vi "Read Keys.vi"(7 "Section":string, 8 "error in (no error)":errorcluster, 10 "Key Names ([]=All Keys)":string[](array[string]), 11 "Config Refnum in":T1) -> (0 "error out":errorcluster, 1 "Values":string[](array[string]), 2 "Key Names":string[](array[string]), 3 "Config Refnum out":T1, 4 "Found":bool[](array[boolean]))   [LabVIEW 2018, in "Core.lvlib" / "Config.lvlib"]
uses:
  Config.lvlib
  <vilib>/Utility/config.llb/NI_LVConfig.lvlib
  <vilib>/Utility/config.llb/Read Key (String).vi
  <vilib>/Utility/config.llb/Config Data RefNum.ctl
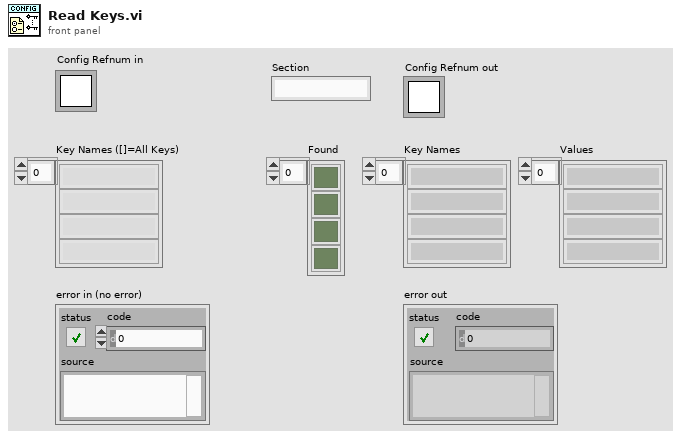
[diagram p1: front panel]
types:
  T1 = typedef "NI_LVConfig.lvlib/Config Data RefNum.ctl" = refnum<k1>
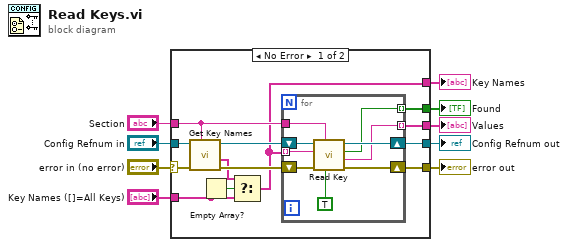
[diagram p0: block diagram]
diagram:
  n1 = case shown="No Error" "error in (no error)" {
    selector: "error in (no error)" -> [w12 w33]
    tunnel: "Section" -> [w20 _]
    tunnel: [w11 w33] -> w7
    tunnel: [w19 _] -> w6
    tunnel: [w18 _] -> w5
    tunnel: "Key Names ([]=All Keys)" -> [w16 _]
    tunnel: [w14 _] -> w3
    tunnel: "Config Refnum in" -> [w13 w32]
    tunnel: [w10 w32] -> w1
    frame No Error {
      n2 = call <vilib>:"Get Key Names.vi"("section"=w20, "error in (no error)"=w12, "refnum"=w13) -> ("error out"=w22:errorcluster, "key names"=w15:string[], "refnum out"=w21:T1)  [unwired: 5 in, 1 out]
      n3 = Empty Array?(array=w16) -> (empty?=w17:bool)
      n4 = Select(t=w15, s=w17, f=w16) -> (s? t:f=w14:string[])
      n5 = for {
        shift-right: [w28] -> w11
        shift-left: w22 -> [w31]
        shift-right: [w29] -> w10
        shift-left: w21 -> [w30]
        tunnel: w14 -> [w26] mode=indexing
        tunnel: w20 -> [w25]
        tunnel: [w24] -> w19 mode=indexing
        tunnel: [w23] -> w18 mode=indexing
        n6 = call-poly <vilib>:"Read Key.vi"("read raw string? (F)"=TRUE, "section"=w25, "error in (no error)"=w31, "key"=w26, "refnum"=w30) -> ("error out"=w28:errorcluster, "value"=w24:string, "found?"=w23:bool, "refnum out"=w29:T1)  [unwired: 3 in]
      }
    }
    frame Error {
    }
  }
  "error out" <- w7
  "Key Names" <- w3
  "Values" <- w6
  "Found" <- w5
  "Config Refnum out" <- w1
